vi "Join Layers.vi"(5 "Locked?":bool, 6 "Rotate? (T)":bool=TRUE, 7 "Active Layer":i32, 9 "User Layers":refnum<class "Layer.lvclass">[](array[class]), 10 "Template":refnum<class "Layer.lvclass">, 11 "Icon Text":refnum<class "Layer.lvclass">) -> (3 "Layer out":refnum<class "Layer.lvclass">[](array[class]))   [LabVIEW 2020, in "lv_icon.lvlib"]
doc: "Joins the Template, Text and User Layers in the right order."
uses:
  <vilib>/LabVIEW Icon API/lv_icon/lv_icon.lvlib
  <vilib>/LabVIEW Icon API/lv_icon/Classes/Layer/Layer.lvclass
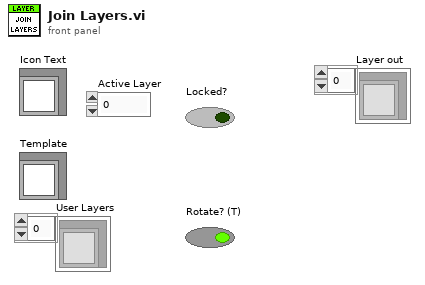
[diagram p1: front panel]
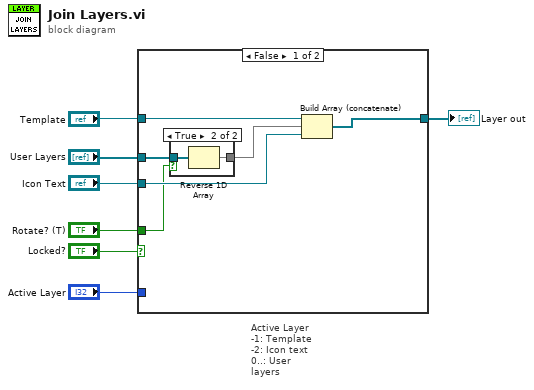
[diagram p0: block diagram]
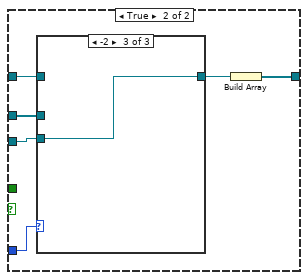
[diagram p3: hidden frame]
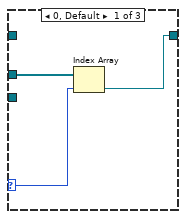
[diagram p4: hidden frame]
diagram:
  # "Active Layer\n-1: Template\n-2: Icon text\n0..: User layers"
  n1 = case shown="False" "Locked?" {
    tunnel: "Template" -> [w12 w21]
    tunnel: "User Layers" -> [w13 w17]
    tunnel: "Icon Text" -> [w10 w20]
    tunnel: [w9 w18] -> w5
    tunnel: "Active Layer" -> [_ w22]
    tunnel: "Rotate? (T)" -> [w8 _]
    frame False {
      n2 = case shown="True" w8 {
        tunnel: w13 -> [w14 w16]
        tunnel: [w14 w15] -> w11
        frame False {
        }
        frame True {
          n3 = Reverse 1D Array(array=w16) -> (reversed array=w15:refnum<class "Layer.lvclass">[])
        }
      }
      n4 = Build Array (concatenate)(w12, w11, w10) -> (w9:refnum<class "Layer.lvclass">[])
    }
    frame True {
      n5 = case shown="-2" w22 {
        selector: w22 -> [w24 _ _]
        tunnel: [w23 w26 w27] -> w19
        tunnel: w21 -> [_ w26 _]
        tunnel: w20 -> [_ _ w27]
        tunnel: w17 -> [w25 _ _]
        frame 0, Default {
          n6 = Index Array(array=w25, index=w24) -> (element=w23:refnum<class "Layer.lvclass">)
        }
        frame -1 {
        }
        frame -2 {
        }
      }
      n7 = Build Array(w19) -> (w18:refnum<class "Layer.lvclass">[])
    }
  }
  "Layer out" <- w5
